vi "ix [SGL].vi"(1 "x (1)":sgl[](array[numeric])) -> (0 "i.(x)":csg[](array[numeric]))   [LabVIEW 2021, in "Math.lvlib"]
doc: "input numeric (default: 1) multiplied by i (complex root of -1)\n\nDepending on what numeric type (optional) is provided, a different type (CXT, CDB or CSG) is returned.\nDefault is Complex Double (CDB)."
uses:
  Math.lvlib
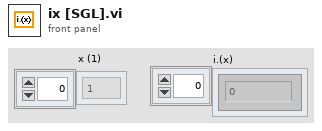
[diagram p1: front panel]
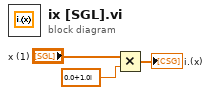
[diagram p0: block diagram]
diagram:
  n1 = Multiply(x="x (1)", y=csg 0.0+1.0i ("i")) -> (x*y=→"i.(x)":csg[])
